vi "Write Query.vi"(8 "error in (no error)":errorcluster, 10 "Query":cluster{"argument":string, "value":string}[](array[cluster]), 11 "URI in":refnum<class "URI.lvclass">) -> (0 "error out":errorcluster, 3 "URI out":refnum<class "URI.lvclass">)   [LabVIEW 2013, in "openURI.lvlib" / "URI.lvclass"]
uses:
  URI.lvclass
  URI.lvclass/URI.ctl
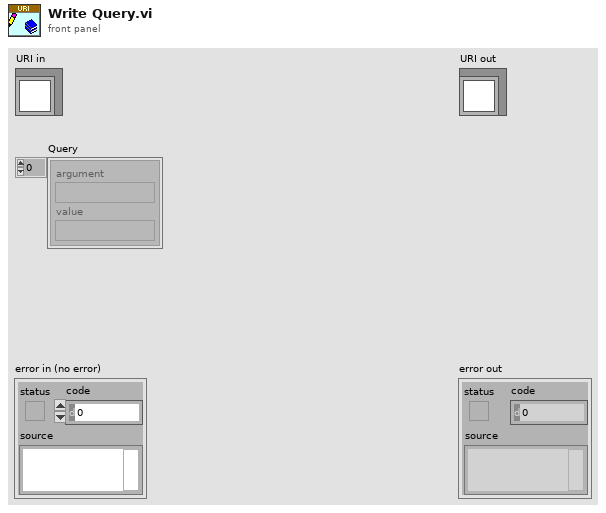
[diagram p1: front panel]
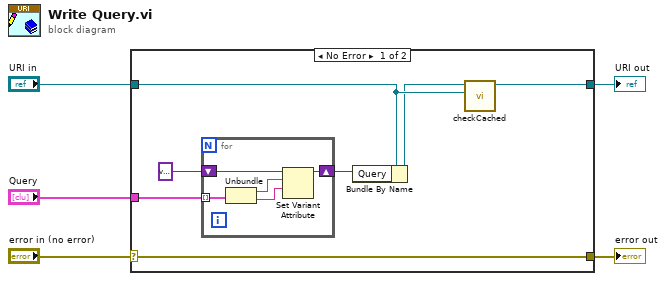
[diagram p0: block diagram]
diagram:
  n1 = case shown="No Error" "error in (no error)" {
    selector: "error in (no error)" -> [w12 w18]
    tunnel: [w12 w18] -> w4
    tunnel: [w9 w19] -> w2
    tunnel: "URI in" -> [w11 w19]
    tunnel: "Query" -> [w6 _]
    frame No Error {
      n2 = for {
        shift-right: [w16] -> w7
        shift-left: variant ("variant") -> [w17]
        tunnel: w6 -> [w15] mode=indexing
        n3 = Unbundle(w15) -> ("argument"=w14:string, "value"=w13:string)
        n4 = Set Variant Attribute(Variant=w17, name=w14, value=w13) -> (Variant out=w16:variant)  [unwired: 1 in, 2 out]
      }
      n5 = Bundle By Name(cluster=w11, "Query"=w7) -> (w10:refnum<class "URI.lvclass">)
      n6 = call "checkCached.vi"("Old"=w11, "New URI"=w10) -> ("URI"=w9:refnum<class "URI.lvclass">)  [unwired: 9 in]
    }
    frame Error {
    }
  }
  "error out" <- w4
  "URI out" <- w2
